vi "GetEdwardsPressureFromVI.vi"(4 "error in":errorcluster) -> (0 "error out":errorcluster, 1 "Boolean":bool, 2 "Volt out":dbl[](array[numeric]), 3 "VI Refnum":refnum<vi>)   [LabVIEW 2019]
panel:
  out "Control Value:Get":variant
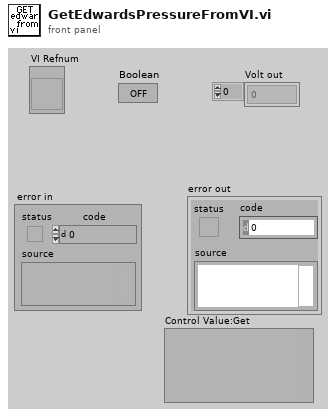
[diagram p1: front panel]
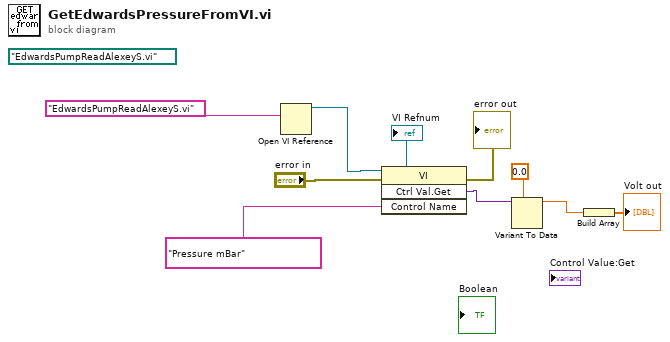
[diagram p0: block diagram]
diagram:
  (unwired) path "EdwardsPumpReadAlexeyS.vi" ("vi path")
  n1 = Open VI Reference(vi path="EdwardsPumpReadAlexeyS.vi" ("Control Name")) -> (vi reference=w7:refnum<vi>)  [unwired: 5 in, 1 out]
  n2 = invoke class="VI" method="Ctrl Val.Get"(reference=w7, error in="error in", "Control Name"="Pressure mBar") -> (reference out=→"VI Refnum":refnum<vi>, error out=→"error out":errorcluster, "Get Control Value Variant"=w2:variant)  [unwired: 1 in, 1 out]
  n3 = Variant To Data(type=0.0, Variant=w2) -> (data=w3:dbl)  [unwired: 1 in, 1 out]
  n4 = Build Array(w3) -> (→"Volt out":dbl[])
